vi "setTimeout.vi"(8 "error in (no error)":errorcluster, 10 "timeout":i32, 11 "Cliente in":refnum<class "Cliente.lvclass">) -> (0 "error out":errorcluster, 3 "Cliente out":refnum<class "Cliente.lvclass">)   [LabVIEW 2015, in "Cliente.lvclass"]
uses:
  Cliente.lvclass
  Cliente.lvclass/Cliente.ctl
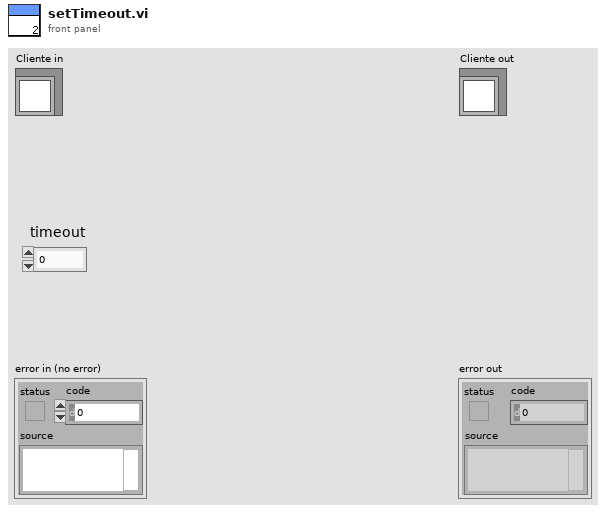
[diagram p1: front panel]
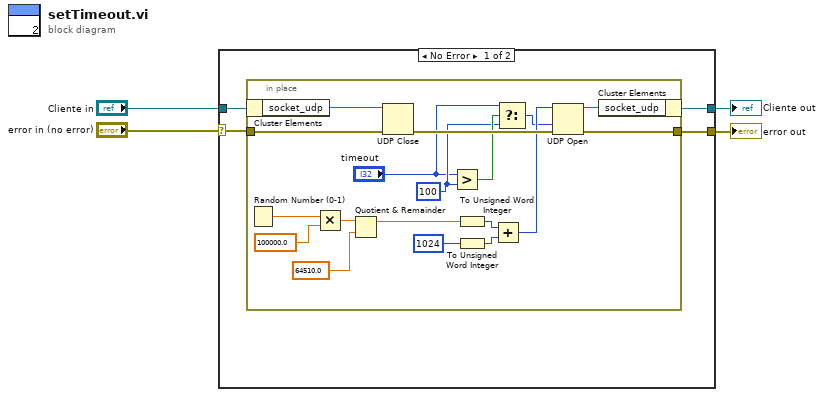
[diagram p0: block diagram]
diagram:
  n1 = case shown="No Error" "error in (no error)" {
    selector: "error in (no error)" -> [w7 w28]
    tunnel: [w6 w28] -> w3
    tunnel: [w5 w27] -> w1
    tunnel: "Cliente in" -> [w8 w27]
    frame No Error {
      n2 = in-place {
        in-place-border: w7 -> [w25]
        in-place-border: [w13] -> w6
        w10 = 100 ("y")
        n3 = in-place-cluster #1(w8) -> ("socket_udp"=w26:refnum<k16>)
        n4 = Random Number (0-1)() -> (number: 0 to 1=w16:dbl)
        n5 = Multiply(x=w16, y=100000.0) -> (x*y=w20:dbl)
        n6 = Quotient & Remainder(x=w20, y=64510.0) -> (x-y*floor(x/y)=w21:dbl)  [unwired: 1 out]
        n7 = UDP Close(connection ID=w26, 8:w25) -> (error out=w24:errorcluster)  [unwired: 1 out]
        n8 = Greater?(x="timeout", y=w10) -> (0:w11:bool)
        n9 = To Unsigned Word Integer(number=w21) -> (unsigned 16bit integer=w18:u16)
        n10 = To Unsigned Word Integer(number=u16 1024) -> (unsigned 16bit integer=w19:u16)
        n11 = Add(x=w18, y=w19) -> (x+y=w14:u16)
        n12 = Select(t="timeout", s=w11, f=w10) -> (s? t:f=w12:i32)
        n13 = UDP Open(8:w24, 9:w12, 11:w14) -> (port=w23:refnum<k16>, 0:w13:errorcluster)  [unwired: 2 in, 1 out]
        n14 = in-place-cluster #1("socket_udp"=w23) -> (w5:refnum<class "Cliente.lvclass">)
      }
    }
    frame Error {
    }
  }
  "error out" <- w3
  "Cliente out" <- w1
